vi "AOTF-Trigger.vi"() -> ()   [LabVIEW 2011]
doc: "I. Description:\nThis example demonstrates how to generate a continuous digital pulse train from a Counter Output Channel started by an external digital trigger. The Frequency, Duty Cycle, and Idle State are all configurable. \n\nThis example shows how to configure the pulse in terms of Frequency/Duty Cycle, but can easily be modified to generate a pulse in terms of Time or Ticks.\n\nII. Instructions for Running:\n1. Select the Physical Channel which corresponds to the counter you want to output your signal to on the DAQ device.\n2. Enter the Frequency and Duty Cycle to define the pulse parameters. You can also change the Idle State to set the state the line will remain in after the generation is stopped. Additionally, you can set the Initial Delay (in seconds) which will delay the beginning of the pulse train from the start call; this is currently wired to 0.0 on the block diagram. \n3. Setup the Trigger Parameters. In this example the VI is expecting a Rising Edge Digital Trigger on PFI9. \n\nIII. Block Diagram Steps:\n1. Create a Counter Output channel to produce a Pulse in terms of Frequency. If the Idle State of the pulse is set to low the first transition of the generated signal is from low to high.\n2. Use the DAQmx Trigger VI to configure a trigger to start on a digital edge.\n2. Use the DAQmx Timing VI (Implicit) to configure the duration of the pulse generation.\n3. Call the Start VI to arm the counter and begin the pulse train generation.\n4. Loop continuously until the user presses the Stop button. Check for errors every 100 ms using the Is Task Done? VI\n5. Call the Clear Task VI to clear the Task.\n\nIV. I/O Connections Overview:\nThe counter will output the pulse train on the output terminal of the counter specified in the Physical Channel I/O control. \n\nIn this example the output will be sent to the default output terminal on ctr0.\n\nFor more information on the default counter input and output terminals for your device, open the NI-DAQmx Help, and refer to Counter Signal Connections found under the Device Considerations book in the table of contents."
uses:
  <vilib>/Utility/error.llb/DialogType.ctl
  <vilib>/DAQmx/write.llb/DAQmx Write (Digital Bool 1Line 1Point).vi
  <vilib>/DAQmx/read.llb/DAQmx Read (Digital Bool 1Line 1Point).vi
  <vilib>/DAQmx/create/channels.llb/DAQmx Create Channel (DI-Digital Input).vi
  <vilib>/DAQmx/create/channels.llb/DAQmx Create Channel (DO-Digital Output).vi
  <vilib>/DAQmx/miscellaneous.llb/DAQmx Fill In Error Info.vi
  <vilib>/DAQmx/create/channels.llb/DAQmx Create Channel (CO-Pulse Generation-Frequency).vi
  <vilib>/DAQmx/configure/trigger.llb/DAQmx Start Trigger (Digital Edge).vi
  <vilib>/DAQmx/configure/timing.llb/DAQmx Timing (Implicit).vi
  Program Files (x86)/National Instruments/LabVIEW 2011/resource/objmgr/daqmx.rc
panel:
  in  "Triggered":bool=TRUE
  out "Delay":dbl[](array[numeric])
  out "Duty cycle":dbl[](array[numeric])
  in  "Pulse length":i16[](array[numeric])
  in  "Sync trigger ratio":i32
  in  "Channel":string="12"
  # "Channel Parameters"
  # "Trigger Parameters"
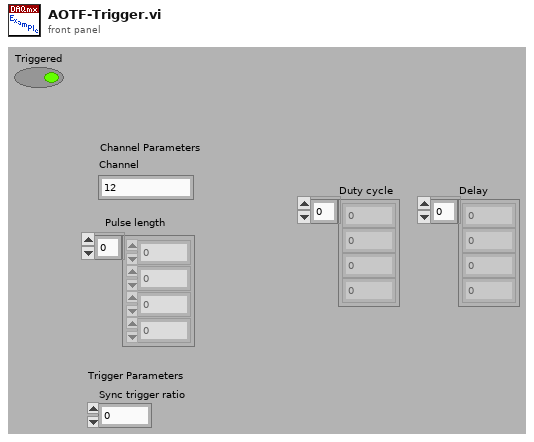
[diagram p1: front panel]
types:
  T1 = typedef "DialogType.ctl" = u16
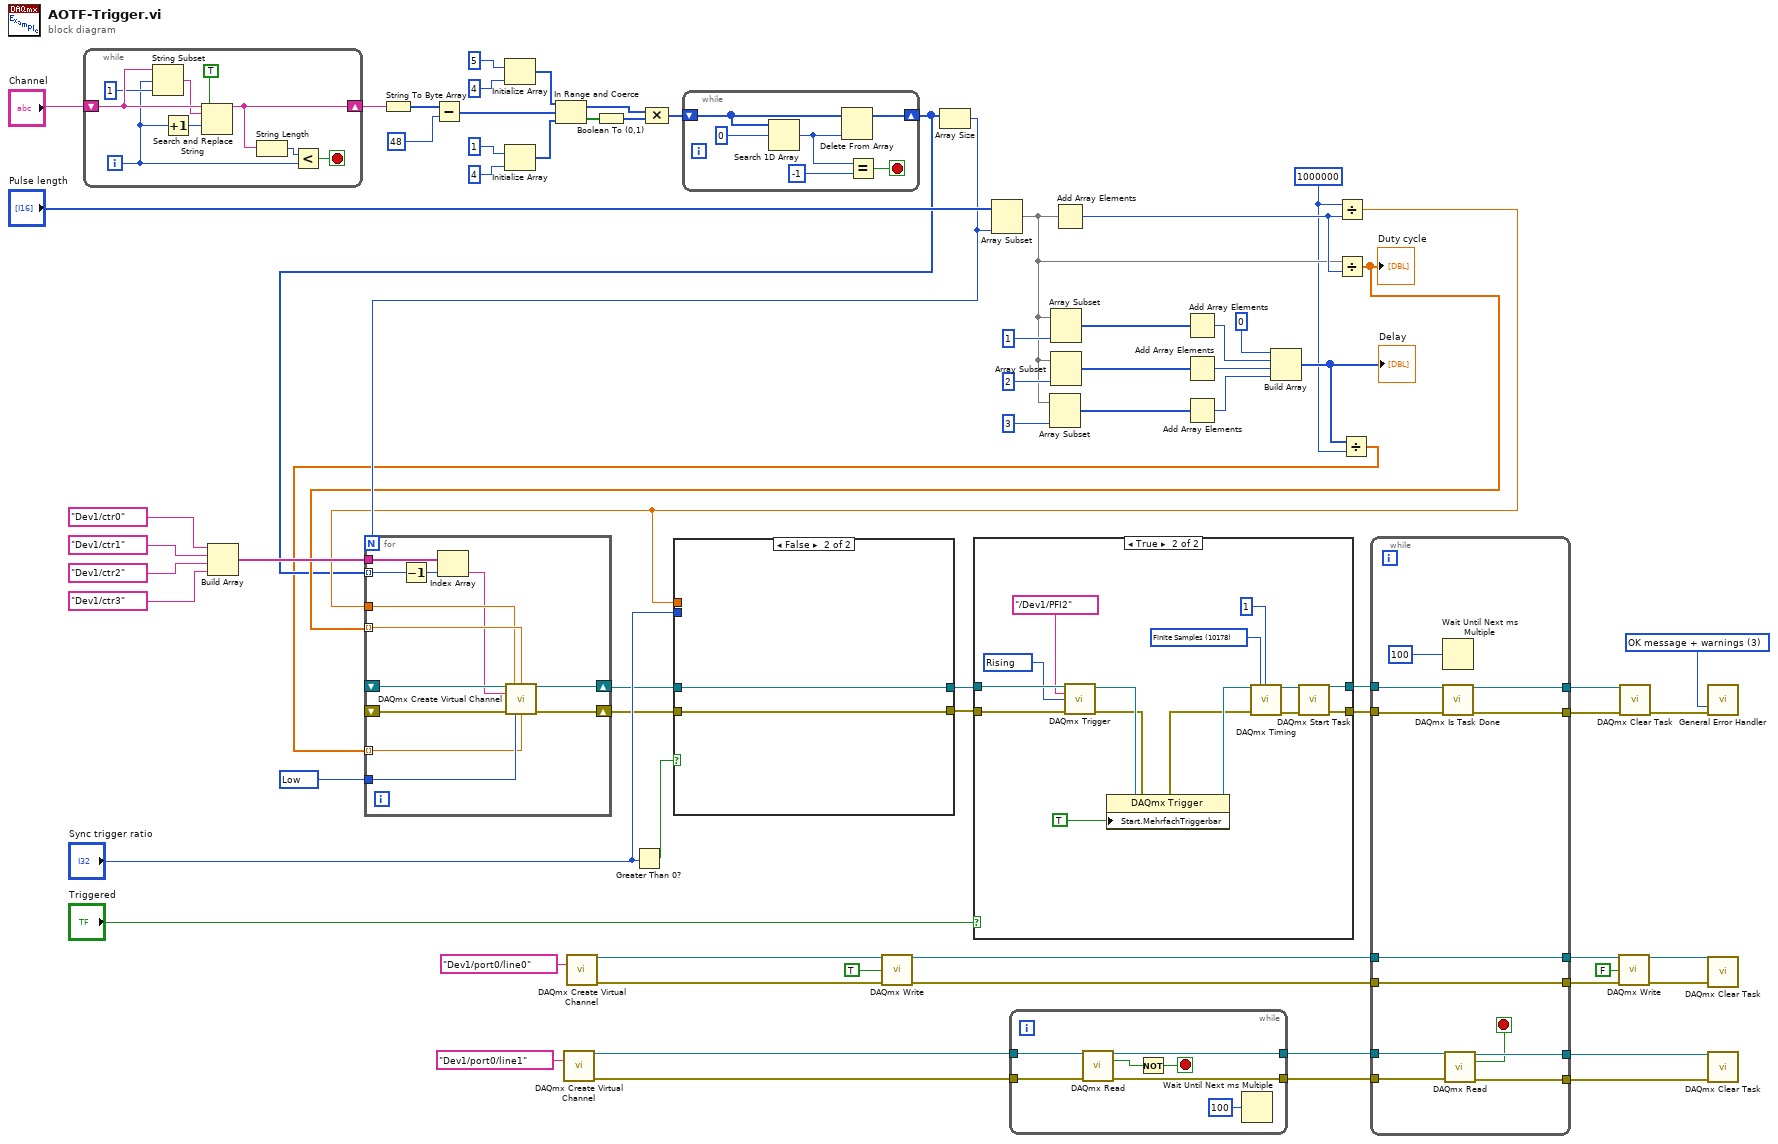
[diagram p0: block diagram]
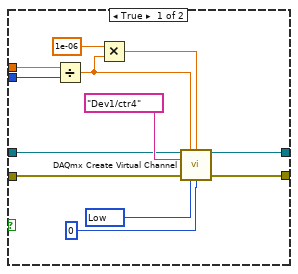
[diagram p2: hidden frame]
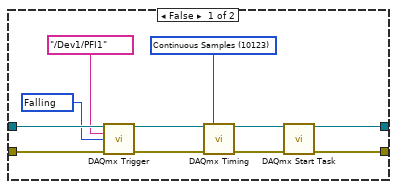
[diagram p3: hidden frame]
diagram:
  w32 = T1 3 items=["no dialog", "OK message", "continue or stop message", "OK message + warnings", "continue/stop + warnings"] ("type of dialog (OK msg:1)")
  w34 = 1000000
  w40 = 10214 items=["High"=10192, "Low"=10214] ("Idle State 2")
  n1 = while {
    shift-right: [w77] -> w61
    shift-left: "Channel" -> [w81]
    i -> [w73]
    stop <- w76 stop-if-true
    n2 = String Subset(string=w81, offset (0)=w73, length (rest)=1) -> (substring=w79:string)
    n3 = Increment(x=w73) -> (x+1=w74:i32)
    n4 = Search and Replace String(replace all?=TRUE, input string=w81, search string=w79, offset=w74) -> (result string=w77:string)  [unwired: 4 in, 3 out]
    n5 = String Length(string=w77) -> (length=w75:i32)
    n6 = Less?(x=w75, y=w73) -> (x < y?=w76:bool)
  }
  n7 = Build Array(tag "Dev1/ctr0" ("Counter 2"), tag "Dev1/ctr1" ("Counter 2"), tag "Dev1/ctr2" ("Counter 2"), tag "Dev1/ctr3" ("Counter 2")) -> (w39:tag[])
  n8 = String To Byte Array(string=w61) -> (unsigned byte array=w64:u8[])
  n9 = Subtract(x=w64, y=48) -> (x-y=w60:i32[])
  n10 = Initialize Array(5, 4) -> (w69:i32[])
  n11 = Initialize Array(1, 4) -> (w66:i32[])
  n12 = In Range and Coerce(upper limit=w69, x=w60, lower limit=w66) -> (coerced(x)=w57:i32[], In Range?=w65:bool[])
  n13 = call-poly <vilib>:"DAQmx Create Virtual Channel.vi"("lines"=tag "Dev1/port0/line1" ("Counter 2")) -> ("task out"=w8:refnum<k21>, "error out"=w7:errorcluster)  [unwired: 13 in]
  n14 = call-poly <vilib>:"DAQmx Create Virtual Channel.vi"("lines"=tag "Dev1/port0/line0" ("Counter 2")) -> ("task out"=w3:refnum<k21>, "error out"=w4:errorcluster)  [unwired: 13 in]
  n15 = Boolean To (0,1)(Boolean=w65) -> (0, 1=w58:i16[])
  n16 = Greater Than 0?(x="Sync trigger ratio") -> (x > 0?=w31:bool)
  n17 = Compound Arithmetic op=MULTIPLY(w57, w58) -> (w59:i32[])
  n18 = while {
    shift-right: [w84] -> w2
    shift-left: w59 -> [w82]
    stop <- w85 stop-if-true
    n19 = Search 1D Array(1D array=w82, element=0) -> (index of element=w86:i32)  [unwired: 1 in]
    n20 = Delete From Array(array=w82, index=w86) -> (array with subset deleted=w84:i32[])  [unwired: 1 in, 1 out]
    n21 = Equal?(x=w86, y=-1) -> (x = y?=w85:bool)
  }
  n22 = call-poly <vilib>:"DAQmx Write.vi"("task/channels in"=w3, "data"=TRUE, "error in"=w4) -> ("task out"=w11:refnum<k21>, "error out"=w12:errorcluster)  [unwired: 10 in, 1 out]
  n23 = Array Size(array=w2) -> (size(s)=w41:i32)
  n24 = Array Subset(array="Pulse length", length=w41) -> (w36:i16[])  [unwired: 1 in]
  n25 = while {
    tunnel: w8 -> [w94]
    tunnel: w7 -> [w93]
    tunnel: [w92] -> w6
    tunnel: [w91] -> w5
    stop <- w88 stop-if-true
    n26 = call-poly <vilib>:"DAQmx Read.vi"("task/channels in"=w94, "error in"=w93) -> ("task out"=w91:refnum<k21>, "data"=w89:bool, "error out"=w92:errorcluster)  [unwired: 11 in]
    n27 = Not(x=w89) -> (.not. x?=w88:bool)
    n28 = Wait Until Next ms Multiple(millisecond multiple=u32 100) -> ()  [unwired: 1 out]
  }
  n29 = Array Subset(array=w36, length=3) -> (w50:i16[])  [unwired: 1 in]
  n30 = Array Subset(array=w36, length=1) -> (w49:i16[])  [unwired: 1 in]
  n31 = Array Subset(array=w36, length=2) -> (w51:i16[])  [unwired: 1 in]
  n32 = Add Array Elements(numeric array=w36) -> (sum=w37:i16)
  n33 = Add Array Elements(numeric array=w49) -> (sum=w46:i16)
  n34 = Add Array Elements(numeric array=w51) -> (sum=w48:i16)
  n35 = Add Array Elements(numeric array=w50) -> (sum=w47:i16)
  n36 = Build Array(0, w46, w48, w47) -> (w35:i32[])
  "Delay" <- w35
  n37 = Divide(x=w34, y=w37) -> (x/y=w25:dbl)
  n38 = Divide(x=w36, y=w37) -> (x/y=w38:dbl[])
  "Duty cycle" <- w38
  n39 = Divide(x=w35, y=w34) -> (x/y=w1:dbl[])
  n40 = for {
    N: w41 -> [_]
    shift-right: [w106] -> w27
    shift-left: _ -> [w105]
    shift-right: [w104] -> w26
    shift-left: _ -> [w103]
    tunnel: w40 -> [w102]
    tunnel: w38 -> [w101] mode=indexing
    tunnel: w25 -> [w100]
    tunnel: w1 -> [w99] mode=indexing
    tunnel: w39 -> [w97]
    tunnel: w2 -> [w96] mode=indexing
    n41 = Decrement(x=w96) -> (x-1=w95:i32)
    n42 = Index Array(array=w97, index=w95) -> (element=w98:tag)
    n43 = call-poly <vilib>:"DAQmx Create Virtual Channel.vi"("task in"=w103, "frequency"=w100, "duty cycle"=w101, "counter"=w98, "error in"=w105, "idle state"=w102, "initial delay"=w99) -> ("task out"=w104:refnum<k21>, "error out"=w106:errorcluster)  [unwired: 7 in]
  }
  n44 = case shown="False" w31 {
    tunnel: [w117 w120] -> w28
    tunnel: [w114 w119] -> w29
    tunnel: w25 -> [w113 _]
    tunnel: "Sync trigger ratio" -> [w112 _]
    tunnel: w27 -> [w108 w119]
    tunnel: w26 -> [w107 w120]
    frame True {
      w115 = 10214 items=["High"=10192, "Low"=10214] ("Idle State 2")
      n45 = Divide(x=w113, y=w112) -> (x/y=w109:dbl)
      n46 = Multiply(x=1e-06, y=w109) -> (x*y=w111:dbl)
      n47 = call-poly <vilib>:"DAQmx Create Virtual Channel.vi"("task in"=w107, "frequency"=w109, "duty cycle"=w111, "counter"=tag "Dev1/ctr4" ("Counter 2"), "error in"=w108, "idle state"=w115, "initial delay"=0) -> ("task out"=w117:refnum<k21>, "error out"=w114:errorcluster)  [unwired: 7 in]
    }
    frame False {
    }
  }
  n48 = case shown="True" "Triggered" {
    tunnel: w29 -> [w128 w143]
    tunnel: w28 -> [w127 w142]
    tunnel: [w124 w138] -> w22
    tunnel: [w123 w137] -> w21
    frame False {
      w125 = u16 10171 items=["Falling"=10171, "Rising"=10280]
      w129 = 10123 items=["Finite Samples"=10178, "Continuous Samples"=10123] ("sample mode")
      n49 = call-poly <vilib>:"DAQmx Trigger.vi"("task/channels in"=w127, "source"=tag "/Dev1/PFI1" ("Trigger Source"), "edge"=w125, "error in"=w128) -> ("task out"=w121:refnum<k21>, "error out"=w122:errorcluster)  [unwired: 10 in]
      n50 = call-poly <vilib>:"DAQmx Timing.vi"("task/channels in"=w121, "sample mode"=w129, "error in"=w122) -> ("task out"=w130:refnum<k21>, "error out"=w131:errorcluster)  [unwired: 11 in]
      n51 = call <vilib>:"DAQmx Start Task.vi"("task/channels in"=w130, "error in"=w131) -> ("task out"=w123:refnum<k21>, "error out"=w124:errorcluster)  [unwired: 12 in]
    }
    frame True {
      w140 = u16 10280 items=["Falling"=10171, "Rising"=10280]
      w144 = 10178 items=["Finite Samples"=10178, "Continuous Samples"=10123] ("sample mode")
      n52 = call-poly <vilib>:"DAQmx Trigger.vi"("task/channels in"=w142, "source"=tag "/Dev1/PFI2" ("Trigger Source"), "edge"=w140, "error in"=w143) -> ("task out"=w135:refnum<k21>, "error out"=w133:errorcluster)  [unwired: 10 in]
      n53 = property class="DAQmx Trigger"(reference=w135, error in=w133, "Start.MehrfachTriggerbar"=TRUE) -> (reference out=w134:refnum<k21>, error out=w132:errorcluster)
      n54 = call-poly <vilib>:"DAQmx Timing.vi"("task/channels in"=w134, "sample mode"=w144, "samples per channel"=1, "error in"=w132) -> ("task out"=w145:refnum<k21>, "error out"=w146:errorcluster)  [unwired: 10 in]
      n55 = call <vilib>:"DAQmx Start Task.vi"("task/channels in"=w145, "error in"=w146) -> ("task out"=w137:refnum<k21>, "error out"=w138:errorcluster)  [unwired: 12 in]
    }
  }
  n56 = while {
    tunnel: w22 -> [w157]
    tunnel: w21 -> [w158]
    tunnel: [w156] -> w23
    tunnel: [w155] -> w24
    tunnel: w5 -> [w151]
    tunnel: w6 -> [w150]
    tunnel: [w147] -> w16
    tunnel: [w148] -> w15
    tunnel: w11 -> [w148]
    tunnel: w12 -> [w147]
    tunnel: [w153] -> w9
    tunnel: [w152] -> w10
    stop <- w149 stop-if-true
    n57 = Wait Until Next ms Multiple(millisecond multiple=u32 100) -> ()  [unwired: 1 out]
    n58 = call <vilib>:"DAQmx Is Task Done.vi"("task/channels in"=w158, "error in"=w157) -> ("task out"=w156:refnum<k21>, "error out"=w155:errorcluster)  [unwired: 11 in, 1 out]
    n59 = call-poly <vilib>:"DAQmx Read.vi"("task/channels in"=w151, "error in"=w150) -> ("task out"=w152:refnum<k21>, "data"=w149:bool, "error out"=w153:errorcluster)  [unwired: 11 in]
  }
  n60 = call-poly <vilib>:"DAQmx Write.vi"("task/channels in"=w15, "data"=FALSE, "error in"=w16) -> ("task out"=w18:refnum<k21>, "error out"=w17:errorcluster)  [unwired: 10 in, 1 out]
  n61 = call <vilib>:"DAQmx Clear Task.vi"("task in"=w23, "error in"=w24) -> ("error out"=w72:errorcluster)  [unwired: 13 in]
  n62 = call <vilib>:"General Error Handler.vi"("type of dialog (OK msg:1)"=w32, "error in (no error)"=w72) -> ()  [unwired: 9 in, 5 out]
  n63 = call <vilib>:"DAQmx Clear Task.vi"("task in"=w18, "error in"=w17) -> ()  [unwired: 13 in, 1 out]
  n64 = call <vilib>:"DAQmx Clear Task.vi"("task in"=w10, "error in"=w9) -> ()  [unwired: 13 in, 1 out]
